vi "SearchRepeatingArray.vi"(0 "Input(ary)":string[](array[string]), 7 "Input(str) empty for array":string) -> (2 "All Words":string[](array[string]), 4 "Statistics":cluster{"times":i32, "Word":string}[](array[cluster]), 6 "No Of Unique Words":i32, 10 "No Of Words":i32)   [LabVIEW 2018]
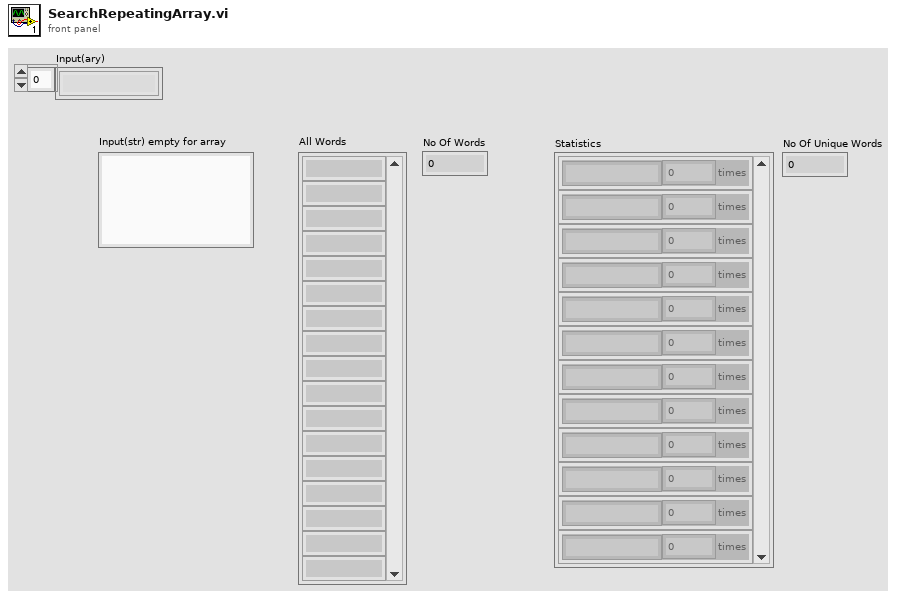
[diagram p1: front panel]
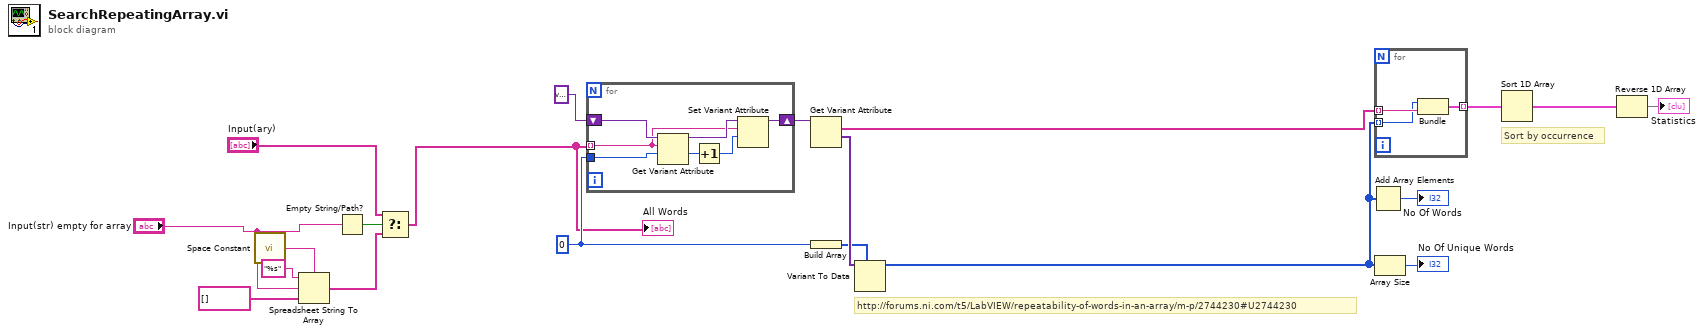
[diagram p0: block diagram]
diagram:
  w6 = 0
  # "http://forums.ni.com/t5/LabVIEW/repeatability-of-words-in-an-array/m-p/2744230#U2744230"
  # "Sort by occurrence"
  n1 = call <vilib>:"Space Constant.vi"() -> ("String"=w18:string)
  n2 = Spreadsheet String To Array(delimiter (Tab)=w18, format string="%s", spreadsheet string="Input(str) empty for array", array type (2D Dbl)=string[] []) -> (array=w4:string[])
  n3 = Empty String/Path?(string/path="Input(str) empty for array") -> (empty?=w2:bool)
  n4 = Select(t="Input(ary)", s=w2, f=w4) -> (s? t:f=w3:string[])
  "All Words" <- w3
  n5 = for {
    tunnel: w3 -> [w21] mode=indexing
    shift-right: [w26] -> w7
    shift-left: variant -> [w27]
    tunnel: w6 -> [w22]
    n6 = Get Variant Attribute(Variant=w27, name=w21, default value (empty Variant)=w22) -> (duplicate Variant=w25:variant, value=w24:i32)  [unwired: 1 in, 2 out]
    n7 = Increment(x=w24) -> (x+1=w23:i32)
    n8 = Set Variant Attribute(Variant=w25, name=w21, value=w23) -> (Variant out=w26:variant)  [unwired: 1 in, 2 out]
  }
  n9 = Get Variant Attribute(Variant=w7) -> (names=w16:string[], values=w15:variant[])  [unwired: 3 in, 2 out]
  n10 = Build Array(w6) -> (w14:i32[])
  n11 = Variant To Data(type=w14, Variant=w15) -> (data=w9:i32[])  [unwired: 1 in, 1 out]
  n12 = Add Array Elements(numeric array=w9) -> (sum=→"No Of Words":i32)
  n13 = for {
    tunnel: w16 -> [w30] mode=indexing
    tunnel: [w29] -> w13 mode=indexing
    tunnel: w9 -> [w28] mode=indexing
    n14 = Bundle(w28, w30) -> (w29:cluster{i32, string})  [unwired: 1 in]
  }
  n15 = Array Size(array=w9) -> (size(s)=→"No Of Unique Words":i32)
  n16 = Sort 1D Array(array=w13) -> (sorted array=w12:cluster{i32, string}[])
  n17 = Reverse 1D Array(array=w12) -> (reversed array=→"Statistics":cluster{i32, string}[])
